vi "PC Take Data With Timer No Objects.vi"(7 "VISA Resource Name In":refnum<visa-resource-name>="GPIB0::23::INSTR", 8 "error in (no error)":errorcluster, 11 "Photon Counter SR 400 in":T1={"Mode"=0, "Count Time"=0.0, "Trigger Frequency"=10000000.0, "Trigger External?"=FALSE, "Gate A Mode"=0, "Gate A Width"=0.0, "Gate A Delay"=0.0, "Gate B Mode"=0, "Gate B Width"=0.0, "Gate B Delay"=0.0} {"Mode" items=["A,B For T Preset", "A-B For T Preset", "A+B For T Preset", "A For B Preset"]; "Gate A Mode" items=["CW", "Fixed"]; "Gate B Mode" items=["CW", "Fixed"]}) -> (0 "error out":errorcluster, 1 "CPS B":dbl[unit], 2 "CPS A":dbl[unit], 3 "Photon counter SR 400 out":T1={"Mode"=0, "Count Time"=0.0, "Trigger Frequency"=10000000.0, "Trigger External?"=FALSE, "Gate A Mode"=0, "Gate A Width"=0.0, "Gate A Delay"=0.0, "Gate B Mode"=0, "Gate B Width"=0.0, "Gate B Delay"=0.0} {"Mode" items=["A,B For T Preset", "A-B For T Preset", "A+B For T Preset", "A For B Preset"]; "Gate A Mode" items=["CW", "Fixed"]; "Gate B Mode" items=["CW", "Fixed"]}, 4 "Counts B":dbl, 5 "VISA Resource Name Out":refnum<visa-resource-name>="GPIB0::23::INSTR", 6 "Counts A":dbl, 10 "Scan Start Time":timestamp)   [LabVIEW 2015]
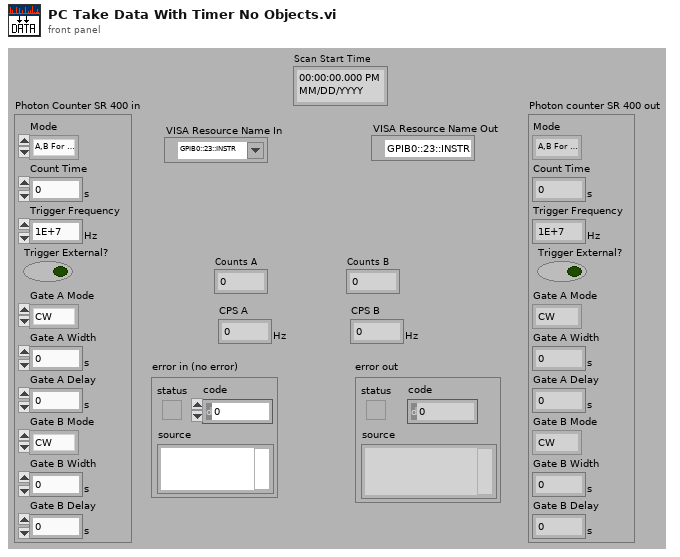
[diagram p1: front panel]
types:
  T1 = cluster{"Mode":u16, "Count Time":dbl[unit], "Trigger Frequency":dbl[unit], "Trigger External?":bool, "Gate A Mode":u16, "Gate A Width":dbl[unit], "Gate A Delay":dbl[unit], "Gate B Mode":u16, "Gate B Width":dbl[unit], "Gate B Delay":dbl[unit]}
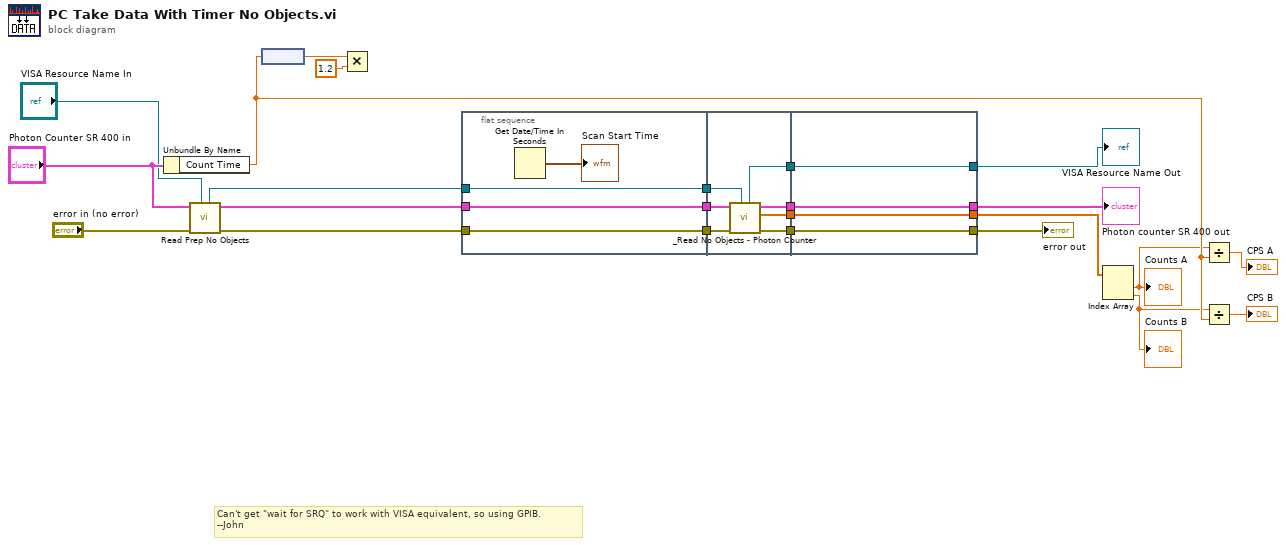
[diagram p0: block diagram]
diagram:
  # "Can't get \"wait for SRQ\" to work with VISA equivalent, so using GPIB. \n--John"
  n1 = Unbundle By Name("Photon Counter SR 400 in") -> ("Count Time"=w24:dbl[unit])
  n2 = call "Read Prep No Objects.vi"("VISA Resource Name In"="VISA Resource Name In", "error in (no error)"="error in (no error)", "Photon Counter SR 400 in"="Photon Counter SR 400 in") -> ("error out"=w3:errorcluster, "Photon Counter SR 400 out"=w12:T1, "VISA Resource Name Out"=w14:refnum<visa-resource-name>)  [unwired: 6 in]
  n3 = node(w24) -> (w22:dbl)
  n4 = Multiply(x=w22, y=1.2) -> ()  [unwired: 1 out]
  n5 = flat-sequence {
    tunnel: w14 -> [w28]
    tunnel: [w28] -> w13
    tunnel: w12 -> [w27]
    tunnel: [w27] -> w11
    tunnel: [w26] -> w10
    tunnel: w3 -> [w26]
    tunnel: w13 -> [w35]
    tunnel: w11 -> [w34]
    tunnel: w10 -> [w33]
    tunnel: [w32] -> w9
    tunnel: [w31] -> w6
    tunnel: [w30] -> w4
    tunnel: [w29] -> w1
    tunnel: w9 -> [w39]
    tunnel: [w39] -> w8
    tunnel: [w38] -> w7
    tunnel: w6 -> [w38]
    tunnel: [w37] -> w5
    tunnel: w4 -> [w37]
    tunnel: [w36] -> w2
    tunnel: w1 -> [w36]
    frame #0 {
      n6 = Get Date/Time In Seconds() -> (seconds since 1Jan1904=→"Scan Start Time":timestamp)
    }
    frame #1 {
      n7 = call "_Read No Objects - Photon Counter.vi"("VISA Resource Name In"=w35, "error in (no error)"=w33, "Photon Counter SR 400 in"=w34) -> ("error out"=w30:errorcluster, "4 Data Points"=w29:dbl[], "Photon Counter SR 400 out"=w32:T1, "VISA Resource Name Out"=w31:refnum<visa-resource-name>)  [unwired: 5 in]
    }
    frame #2 {
    }
  }
  n8 = Index Array(array=w2) -> (element #1=w19:dbl, element #2=w18:dbl)  [unwired: 2 in]
  "Counts B" <- w18
  "Counts A" <- w19
  n9 = Divide(x=w19, y=w24) -> (x/y=→"CPS A":dbl[unit])
  n10 = Divide(x=w18, y=w24) -> (x/y=→"CPS B":dbl[unit])
  "error out" <- w5
  "Photon counter SR 400 out" <- w8
  "VISA Resource Name Out" <- w7
